vi "Launcher.vi"() -> ()   [LabVIEW 2020]
uses:
  UI/UI.lvclass
  C:/Program Files (x86)/National Instruments/LabVIEW 2020/vi.lib/ActorFramework/Actor/Actor.lvclass
  Implementations/Cypress/Cypress.lvclass
  C:/Users/Alex/Documents/ProyectoLabviewFinal/Abstract/Serial Device/Serial Device.lvclass
  Implementations/Simulada/Simulada.lvclass
  Implementations/NXP/NXP.lvclass
  UI/UI.lvclass/UI.ctl
  UI/Write Serial Device.lvclass.vi
  UI/Write Device.vi
  UI/Write VISA resource name.vi
  <vilib>/ActorFramework/Actor/Actor.lvclass
panel:
  in  "VISA resource name":refnum<visa-resource-name>
  in  "Device":enum16{"Cypress", "Simulado", "NXP"}(ring)
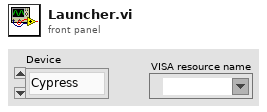
[diagram p1: front panel]
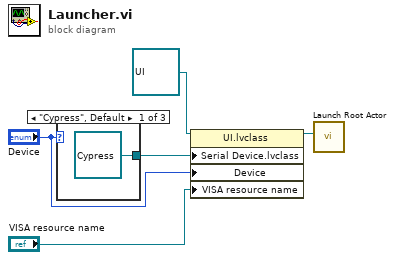
[diagram p0: block diagram]
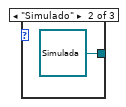
[diagram p2: hidden frame]
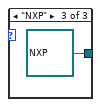
[diagram p3: hidden frame]
diagram:
  n1 = case shown="\"Cypress\", Default" "Device" {
    tunnel: [refnum<class "Cypress.lvclass"> refnum ("Cypress.lvclass") refnum<class "Simulada.lvclass"> refnum ("Simulada.lvclass") refnum<class "NXP.lvclass"> refnum ("NXP.lvclass")] -> w2
    frame "Cypress", Default {
    }
    frame "Simulado" {
    }
    frame "NXP" {
    }
  }
  n2 = property class="UI.lvclass"(reference=refnum<class "UI.lvclass"> refnum ("UI.lvlib:UI.lvclass"), "Serial Device.lvclass"=w2, "Device"="Device", "VISA resource name"="VISA resource name") -> (reference out=w4:refnum<class "UI.lvclass">)  [unwired: 1 in, 1 out]
  n3 = call <vilib>:"Launch Root Actor.vi"("Actor"=w4) -> ()  [unwired: 9 in, 2 out]
